vi "uart_PRIZM.vi"(0 "Motor_Derecho":dbl, 2 "Motor_Izquierdo":dbl, 3 "Motor_Riel":dbl, 5 "Servo_Gripper":dbl) -> (10 "Trama de envío":string, 11 "Trama Recibida":string, 14 "Ultrasonido_1":dbl, 15 "Ultrasonido_2":dbl, 16 "Distancia_ToF":dbl, 17 "Vel_Derecho":dbl, 18 "Vel_Izquierdo":dbl)   [LabVIEW 2019]
uses:
  <vilib>/myRIO/Instrument Drivers/Onboard IO/UART/typedef/VISA Configuration.ctl
  <vilib>/Instr/_visa.llb/VISA Configure Serial Port (Instr).vi
  <vilib>/myRIO/Express VI/Onboard IO/UART/UART Express VI.xnode
  <vilib>/myRIO/Instrument Drivers/Onboard IO/UART/UART.lvlib
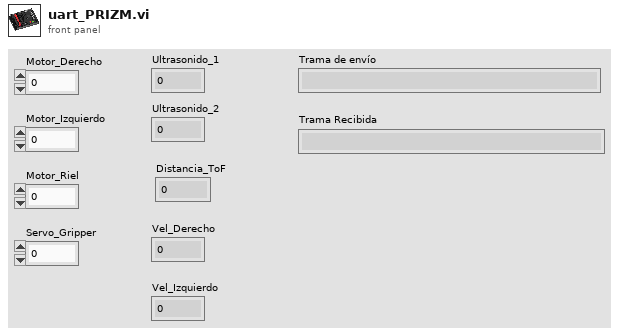
[diagram p1: front panel]
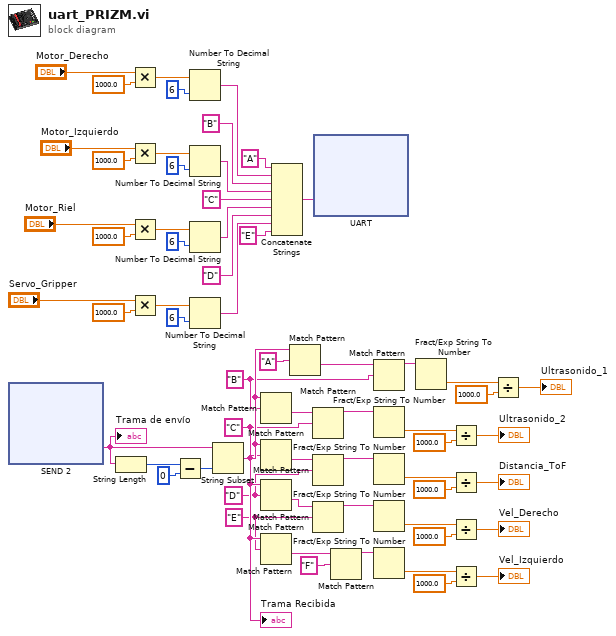
[diagram p0: block diagram]
diagram:
  w34 = "E" ("regular expression")
  w35 = "D" ("regular expression")
  w36 = "C" ("regular expression")
  w37 = "B" ("regular expression")
  n1 = xnode "SEND 2"() -> ("Characters Read"=w1:string)  [unwired: 1 in, 1 out]
  "Trama de envío" <- w1
  n2 = String Length(string=w1) -> (length=w39:i32)
  n3 = Multiply(x="Motor_Derecho", y=1000.0) -> (x*y=w32:dbl)
  n4 = Multiply(x="Motor_Izquierdo", y=1000.0) -> (x*y=w26:dbl)
  n5 = Multiply(x="Motor_Riel", y=1000.0) -> (x*y=w25:dbl)
  n6 = Multiply(x="Servo_Gripper", y=1000.0) -> (x*y=w27:dbl)
  n7 = Subtract(x=w39, y=0) -> (x-y=w41:i32)
  n8 = Number To Decimal String(number=w32, width (-)=i16 6) -> (decimal integer string=w54:string)
  n9 = Number To Decimal String(number=w26, width (-)=i16 6) -> (decimal integer string=w56:string)
  n10 = Number To Decimal String(number=w25, width (-)=i16 6) -> (decimal integer string=w58:string)
  n11 = Number To Decimal String(number=w27, width (-)=i16 6) -> (decimal integer string=w61:string)
  n12 = String Subset(string=w1, length (rest)=w41) -> (substring=w38:string)  [unwired: 1 in]
  "Trama Recibida" <- w38
  n13 = Match Pattern(string=w38, regular expression=w37) -> (after substring=w49:string)  [unwired: 1 in, 3 out]
  n14 = Match Pattern(string=w38, regular expression=w36) -> (after substring=w48:string)  [unwired: 1 in, 3 out]
  n15 = Match Pattern(string=w38, regular expression=w35) -> (after substring=w45:string)  [unwired: 1 in, 3 out]
  n16 = Match Pattern(string=w38, regular expression=w34) -> (after substring=w44:string)  [unwired: 1 in, 3 out]
  n17 = Concatenate Strings("A" ("string"), w54, "B" ("string"), w56, "C" ("string"), w58, "D" ("string"), w61, "E" ("string")) -> (w2:string)
  n18 = Match Pattern(string=w38, regular expression="A") -> (after substring=w53:string)  [unwired: 1 in, 3 out]
  n19 = Match Pattern(string=w49, regular expression=w36) -> (before substring=w50:string)  [unwired: 1 in, 3 out]
  n20 = Match Pattern(string=w48, regular expression=w35) -> (before substring=w47:string)  [unwired: 1 in, 3 out]
  n21 = Match Pattern(string=w45, regular expression=w34) -> (before substring=w46:string)  [unwired: 1 in, 3 out]
  n22 = xnode "UART"("Characters to Write"=w2) -> ()  [unwired: 1 in, 2 out]
  n23 = Match Pattern(string=w44, regular expression="F") -> (before substring=w42:string)  [unwired: 1 in, 3 out]
  n24 = Match Pattern(string=w53, regular expression=w37) -> (before substring=w51:string)  [unwired: 1 in, 3 out]
  n25 = Fract/Exp String To Number(string=w50) -> (number=w10:dbl)  [unwired: 3 in, 1 out]
  n26 = Fract/Exp String To Number(string=w47) -> (number=w9:dbl)  [unwired: 3 in, 1 out]
  n27 = Fract/Exp String To Number(string=w46) -> (number=w8:dbl)  [unwired: 3 in, 1 out]
  n28 = Fract/Exp String To Number(string=w42) -> (number=w7:dbl)  [unwired: 3 in, 1 out]
  n29 = Fract/Exp String To Number(string=w51) -> (number=w16:dbl)  [unwired: 3 in, 1 out]
  n30 = Divide(x=w10, y=1000.0) -> (x/y=→"Ultrasonido_2":dbl)
  n31 = Divide(x=w9, y=1000.0) -> (x/y=→"Distancia_ToF":dbl)
  n32 = Divide(x=w8, y=1000.0) -> (x/y=→"Vel_Derecho":dbl)
  n33 = Divide(x=w7, y=1000.0) -> (x/y=→"Vel_Izquierdo":dbl)
  n34 = Divide(x=w16, y=1000.0) -> (x/y=→"Ultrasonido_1":dbl)
